vi "stopAgent.vi"(8 "error in":errorcluster, 11 "connection ID":refnum<k16>) -> ()   [LabVIEW 2021]
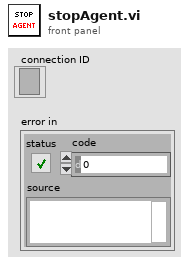
[diagram p1: front panel]
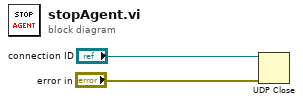
[diagram p0: block diagram]
diagram:
  n1 = UDP Close(connection ID="connection ID", 8:"error in") -> ()  [unwired: 2 out]
